vi "Initiate Autotune.vi"(0 "VISA resource name":refnum<visa-resource-name>, 5 "Output's Control Loop (1:1)":u16(ring)=1 items=["1"=1, "2"=2, "3"=3, "4"=4], 7 "Mode (0:P Only)":u16(ring) items=["P Only", "P and I", "P, I, and D"], 11 "error in (no error)":errorcluster) -> (4 "VISA resource name out":refnum<visa-resource-name>, 15 "error out":errorcluster)   [LabVIEW 2015, in "Lake Shore 350.lvlib"]
doc: "Initiates the Autotune process. Before initiating the Autotune process, the colling system must be configured properly with control input sensor and heater output making it capable of closed-looop cotrol. The control sensor must have a valid temperature response curve assigned to it. An appropriate heater range must also be determined. The system must be coarsely maintaining temperature within 5 k of the setpoint where new tuning parameters are desired in order for the Autotuning process to initiate."
uses:
  Lake Shore 350.lvlib
  Instance           1 25Saved   Initiate Autotune .vi
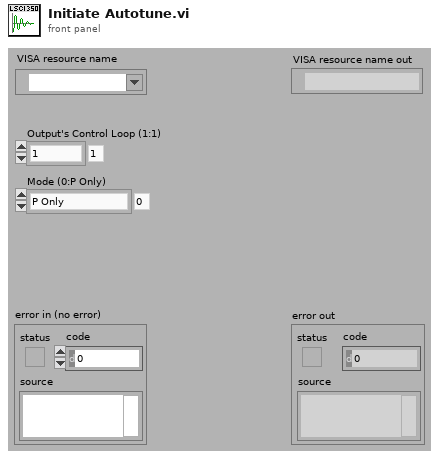
[diagram p1: front panel]
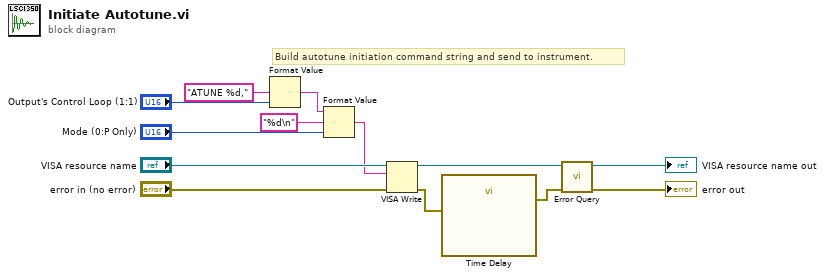
[diagram p0: block diagram]
diagram:
  # "Build autotune initiation command string and send to instrument."
  n1 = Format Value(format string="ATUNE %d,", value (0)="Output's Control Loop (1:1)") -> (output string=w1:string)  [unwired: 1 in]
  n2 = Format Value(string ("")=w1, format string="%d\n", value (0)="Mode (0:P Only)") -> (output string=w4:string)
  n3 = VISA Write(VISA resource name="VISA resource name", write buffer=w4, error in (no error)="error in (no error)") -> (VISA resource name out=w9:refnum<visa-resource-name>, error out=w7:errorcluster)  [unwired: 1 out]
  n4 = call "Time Delay"("error in (no error)"=w7) -> ("error out"=w6:errorcluster)  [unwired: 10 in]
  n5 = call "Error Query.vi"("error in (no error)"=w6, "VISA resource name"=w9) -> ("error out"=→"error out":errorcluster, "VISA resource name out"=→"VISA resource name out":refnum<visa-resource-name>)  [unwired: 7 in, 1 out]
